vi "Rename Window.vi"(4 "error in (no error)":errorcluster, 5 "new window name (\"\")":string, 6 "current window name (\"\")":string, 7 "window refnum (NaWR)":T1) -> (0 "error out":errorcluster, 2 "prev window name":string, 3 "window refnum out":T1)   [LabVIEW 2023, in "WINUTIL.lvlib"]
doc: "This VI will rename the window identified either by its title or by its window refnum. If the window refnum is supplied, the name of the window before renaming is returned in the 'prev window name' output. If the window name is used to identify the window (current window name), then 'prev window name' = 'current window name'."
uses:
  WINUTIL.lvlib
  Window Refnum.ctl
  user32.dll
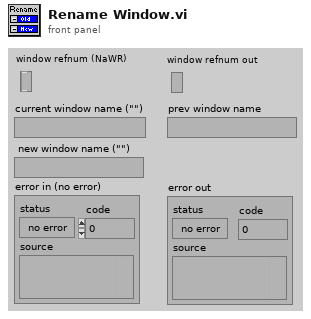
[diagram p1: front panel]
types:
  T1 = typedef "WINUTIL.lvlib/Window Refnum.ctl" = refnum<k1>
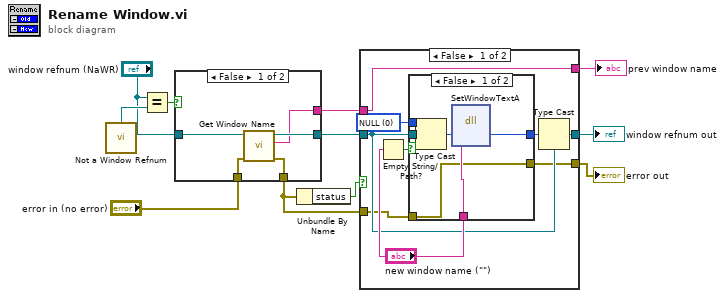
[diagram p0: block diagram]
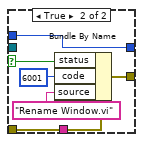
[diagram p2: hidden frame]
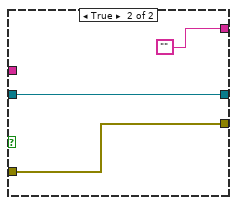
[diagram p3: hidden frame]
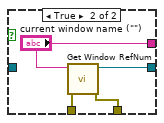
[diagram p4: hidden frame]
diagram:
  n1 = call "Not a Window Refnum.vi"() -> ("Not a Window Refnum"=w5:T1)
  n2 = Equal?(x="window refnum (NaWR)", y=w5) -> (x = y?=w6:bool)
  n3 = case shown="False" w6 {
    tunnel: "error in (no error)" -> [w15 w20]
    tunnel: [w14 w19] -> w2
    tunnel: "window refnum (NaWR)" -> [w16 _]
    tunnel: [w13 w18] -> w10
    tunnel: [w12 "current window name (\"\")"] -> w8
    frame False {
      n4 = call "Get Window Name.vi"("error in (no error)"=w15, "window refnum in (NaWR)"=w16) -> ("error out"=w14:errorcluster, "window name"=w12:string, "window refnum out"=w13:T1)  [unwired: 3 out]
    }
    frame True {
      n5 = call "Get Window RefNum.vi"("error in (no error)"=w20, "window name (\"\")"="current window name (\"\")") -> ("error out"=w19:errorcluster, "window refnum (NaWR)"=w18:T1)  [unwired: 6 out]
    }
  }
  n6 = Unbundle By Name(w2) -> ("status"=w9:bool)
  n7 = case shown="False" w9 {
    tunnel: w10 -> [w23 w43]
    tunnel: [w27 w43] -> w3
    tunnel: w8 -> [w29 _]
    tunnel: [w29 ""] -> w7
    tunnel: w2 -> [w22 w42]
    tunnel: [w21 w42] -> w1
    frame False {
      w24 = u32 0 items=["NULL"]
      n8 = Empty String/Path?(string/path="new window name (\"\")") -> (empty?=w26:bool)
      n9 = case shown="False" w26 {
        selector: w26 -> [_ w37]
        tunnel: w23 -> [w35 _]
        tunnel: [w34 w41] -> w28
        tunnel: "new window name (\"\")" -> [w32 _]
        tunnel: w24 -> [w31 w41]
        tunnel: w22 -> [w30 w39]
        tunnel: [w30 w36] -> w21
        frame False {
          n10 = Type Cast(type=w31, x=w35) -> (*(type *) &x=w33:u32)
          n11 = dll-call lib="USER32.DLL" fn="SetWindowTextA" label="SetWindowText"("hWnd"=w33, "windowName"=w32) -> ("hWnd"=w34:u32)  [unwired: 4 in, 3 out]
        }
        frame True {
          n12 = Bundle By Name(cluster=w39, "status"=w37, "code"=6001, "source"="Rename Window.vi") -> (w36:errorcluster)
        }
      }
      n13 = Type Cast(type=w23, x=w28) -> (*(type *) &x=w27:T1)
    }
    frame True {
    }
  }
  "error out" <- w1
  "prev window name" <- w7
  "window refnum out" <- w3
